vi "DeviceOff.vi"(8 "error in (no error)":errorcluster, 11 "PacificPowerSource in":refnum<class "PacificPowerSource.lvclass">) -> (0 "error out":errorcluster, 3 "PacificPowerSource out":refnum<class "PacificPowerSource.lvclass">)   [LabVIEW 2018, in "AcPwrPlugins.lvlib" / "PacificPowerSource.lvclass"]
doc: "This VI sets the output to off by opening the output switch."
uses:
  PacificPowerSource.lvclass
  <instrlib>/Pacific Power UPC Series/Pacific Power UPC Series.lvlib
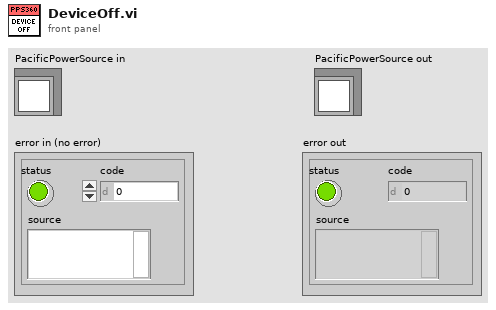
[diagram p1: front panel]
types:
  T1 = typedef "AcPwrPlugins.lvlib/PacificPowerSource.lvclass/DeviceSettings.ctl" = cluster{"Handle":string, "Connected":bool, "Clear Device (F)":bool, "btnIdQuery":bool, "btnReset":bool, "Program #":cluster{"Phase B (Degrees)":i32, "Waveform A (1: Sine)":i32, "Voltage Level (Va)":dbl, "Program Number (0)":i32, "Voltage Level (Vb) ":dbl, "Form (3: Three)":u16, "Coupling  (0: Direct)":u16, "Frequency (45Hz)":dbl, "Current Limit (40A)":dbl, "Phase C (Degrees)":i32, "Voltage Level (Vc)":dbl, "Waveform B (1: Sine)":i32, "Waveform C (1: Sine)":i32}[], "Impedance Parameters (off, 0.00)":cluster{"State":bool, "Impedance":dbl}, "Transient Execution (F)":bool, "OutputEnabled":bool, "Source Range":cluster{"Frequency Minimum (45 Hz)":dbl, "Frequency Maximum (1200 Hz)":dbl, "Voltage Maximum (V)":dbl, "Voltage Minimum (V)":dbl, "Range Control (0: Auto)":u16, "Initial Voltage (0V)":u16, "Frequency Range (600Hz)":u16}, "Port Type":enum16{"GPIB", "Serial"}}[]
  T2 = cluster{"Phase B (Degrees)":i32, "Waveform A (1: Sine)":i32, "Voltage Level (Va)":dbl, "Program Number (0)":i32, "Voltage Level (Vb) ":dbl, "Form (3: Three)":u16, "Coupling  (0: Direct)":u16, "Frequency (45Hz)":dbl, "Current Limit (40A)":dbl, "Phase C (Degrees)":i32, "Voltage Level (Vc)":dbl, "Waveform B (1: Sine)":i32, "Waveform C (1: Sine)":i32}[]
  T3 = cluster{"Phase B (Degrees)":i32, "Waveform A (1: Sine)":i32, "Voltage Level (Va)":dbl, "Program Number (0)":i32, "Voltage Level (Vb) ":dbl, "Form (3: Three)":u16, "Coupling  (0: Direct)":u16, "Frequency (45Hz)":dbl, "Current Limit (40A)":dbl, "Phase C (Degrees)":i32, "Voltage Level (Vc)":dbl, "Waveform B (1: Sine)":i32, "Waveform C (1: Sine)":i32}
  T4 = cluster{"Handle":string, "Connected":bool, "Clear Device (F)":bool, "btnIdQuery":bool, "btnReset":bool, "Program #":cluster{"Phase B (Degrees)":i32, "Waveform A (1: Sine)":i32, "Voltage Level (Va)":dbl, "Program Number (0)":i32, "Voltage Level (Vb) ":dbl, "Form (3: Three)":u16, "Coupling  (0: Direct)":u16, "Frequency (45Hz)":dbl, "Current Limit (40A)":dbl, "Phase C (Degrees)":i32, "Voltage Level (Vc)":dbl, "Waveform B (1: Sine)":i32, "Waveform C (1: Sine)":i32}[], "Impedance Parameters (off, 0.00)":cluster{"State":bool, "Impedance":dbl}, "Transient Execution (F)":bool, "OutputEnabled":bool, "Source Range":cluster{"Frequency Minimum (45 Hz)":dbl, "Frequency Maximum (1200 Hz)":dbl, "Voltage Maximum (V)":dbl, "Voltage Minimum (V)":dbl, "Range Control (0: Auto)":u16, "Initial Voltage (0V)":u16, "Frequency Range (600Hz)":u16}, "Port Type":enum16{"GPIB", "Serial"}}
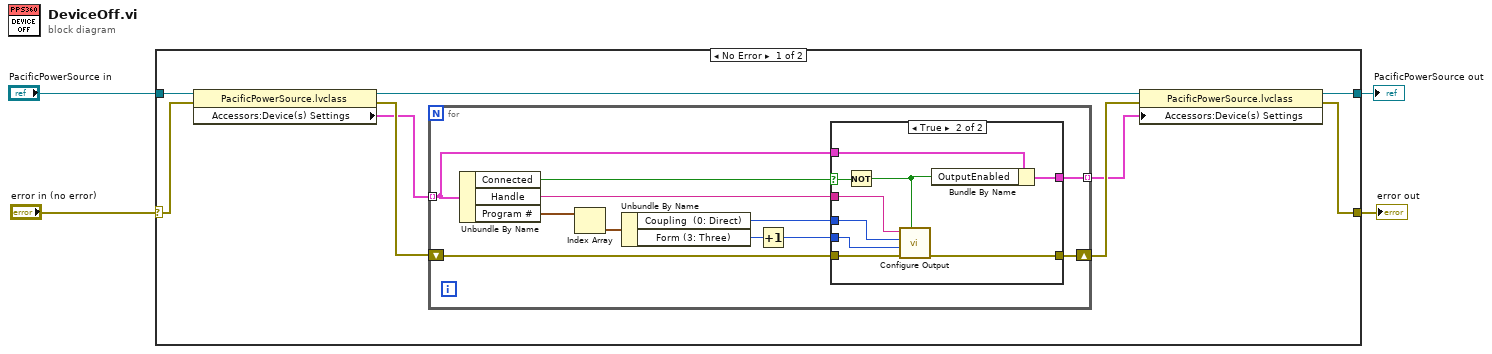
[diagram p0: block diagram]
diagram:
  n1 = case shown="No Error" "error in (no error)" {
    selector: "error in (no error)" -> [w12 w37]
    tunnel: [w7 w37] -> w1
    tunnel: [w8 w36] -> w2
    tunnel: "PacificPowerSource in" -> [w13 w36]
    frame No Error {
      n2 = property class="PacificPowerSource.lvclass"(reference=w13, error in=w12) -> (reference out=w9:refnum<class "PacificPowerSource.lvclass">, error out=w11:errorcluster, "Accessors:Device(s) Settings"=w10:T1)
      n3 = for {
        tunnel: w10 -> [w20] mode=indexing
        shift-right: [w21] -> w6
        shift-left: w11 -> [w22]
        tunnel: [w19] -> w5 mode=indexing
        n4 = Unbundle By Name(w20) -> ("Connected"=w23:bool, "Handle"=w24:string, "Program #"=w16:T2)
        n5 = Index Array(array=w16) -> (element=w18:T3)  [unwired: 1 in]
        n6 = Unbundle By Name(w18) -> ("Coupling  (0: Direct)"=w15:u16, "Form (3: Three)"=w17:u16)
        n7 = Increment(x=w17) -> (x+1=w14:u16)
        n8 = case shown="True" w23 {
          selector: w23 -> [_ w33]
          tunnel: w22 -> [w26 w34]
          tunnel: [w26 w35] -> w21
          tunnel: w24 -> [_ w32]
          tunnel: w20 -> [w25 w31]
          tunnel: [w25 w29] -> w19
          tunnel: w15 -> [_ w28]
          tunnel: w14 -> [_ w27]
          frame False {
          }
          frame True {
            n9 = Not(x=w33) -> (.not. x?=w30:bool)
            n10 = call <instrlib>:"Configure Output.vi"("Enable Output (T: Enable)"=w30, "error in (no error)"=w34, "Form (3: Three)"=w27, "Coupling  (0: Direct)"=w28, "VISA resource name"=w32) -> ("error out"=w35:errorcluster)  [unwired: 5 in, 1 out]
            n11 = Bundle By Name(cluster=w31, "OutputEnabled"=w30) -> (w29:T4)
          }
        }
      }
      n12 = property class="PacificPowerSource.lvclass"(reference=w9, error in=w6, "Accessors:Device(s) Settings"=w5) -> (reference out=w8:refnum<class "PacificPowerSource.lvclass">, error out=w7:errorcluster)
    }
    frame Error {
    }
  }
  "error out" <- w1
  "PacificPowerSource out" <- w2
